vi "calibrationElectrometer_logEvent_intensity.vi"(8 "error in (no error)":errorcluster, 11 "logevent_intensity_Ctl":T1={"electId"=0, "intensity"=0.0, "unit"="                                                                                                                                                                                                                                                                ", "timestamp"=0.0, "priority"=0}) -> (0 "error out":errorcluster, 2 "function return":i32, 3 "logevent_intensity_Ctl out":T1={"electId"=0, "intensity"=0.0, "unit"="                                                                                                                                                                                                                                                                ", "timestamp"=0.0, "priority"=0})   [LabVIEW 2016, in "SALLV_calibrationElectrometer.lvlib"]
doc: "int calibrationElectrometer_shm_logEvent_intensityLV(calibrationElectrometer_logevent_intensityLV *logevent_intensity_Ctl );"
uses:
  SALLV_calibrationElectrometer.lvlib
  DataTypes/logevent_intensity.ctl
  SALLV_calibrationElectrometer.so
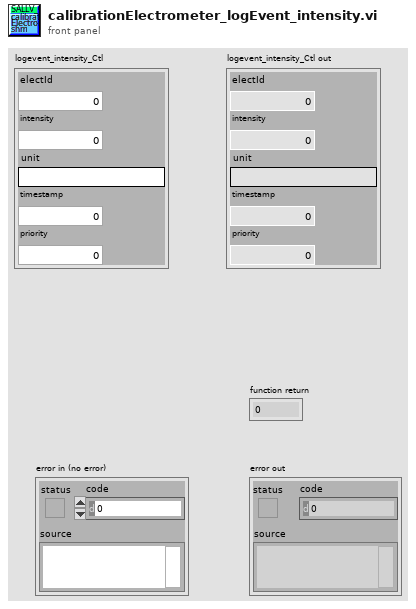
[diagram p1: front panel]
types:
  T1 = typedef "SALLV_calibrationElectrometer.lvlib/logevent_intensity.ctl" = cluster{"electId":i32, "intensity":dbl, "unit":string, "timestamp":dbl, "priority":i32}
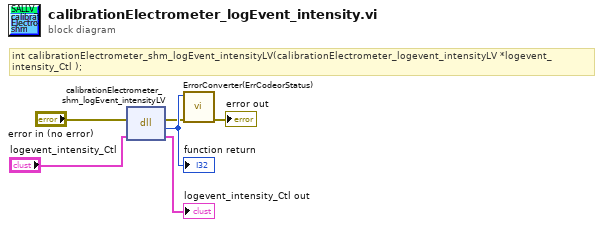
[diagram p0: block diagram]
diagram:
  # "int calibrationElectrometer_shm_logEvent_intensityLV(calibrationElectrometer_logevent_intensityLV *logevent_intensity_Ctl );"
  n1 = dll-call lib="home/andres/Desktop/SAL_calibrationElectrometer/SALLV_calibrationElectrometer.*" fn="calibrationElectrometer_shm_logEvent_intensityLV"(error in="error in (no error)", "logevent_intensity_Ctl"="logevent_intensity_Ctl") -> (error out=w2:errorcluster, w6:i32, "logevent_intensity_Ctl"=→"logevent_intensity_Ctl out":T1)  [unwired: 2 in, 1 out]
  "function return" <- w6
  n2 = call "ErrorConverter(ErrCodeorStatus).vi"("error in (no error)"=w2, "error code"=w6) -> ("error out"=→"error out":errorcluster)  [unwired: 9 in]
